vi "Size.vi"(8 "error in (no error)":errorcluster, 11 "Parameter to Hardware Map in":refnum<class "Parameter to Hardware Map.lvclass">) -> (0 "error out":errorcluster, 2 "Size":i32, 3 "Parameter to Hardware Map out":refnum<class "Parameter to Hardware Map.lvclass">)   [LabVIEW 2020, in "RxnRover.lvlib" / "Parameter to Hardware Map.lvclass"]
doc: "Return the size of the map."
uses:
  Parameter to Hardware Map.lvclass
  Parameter to Hardware Map.lvclass/Parameter to Hardware Map.ctl
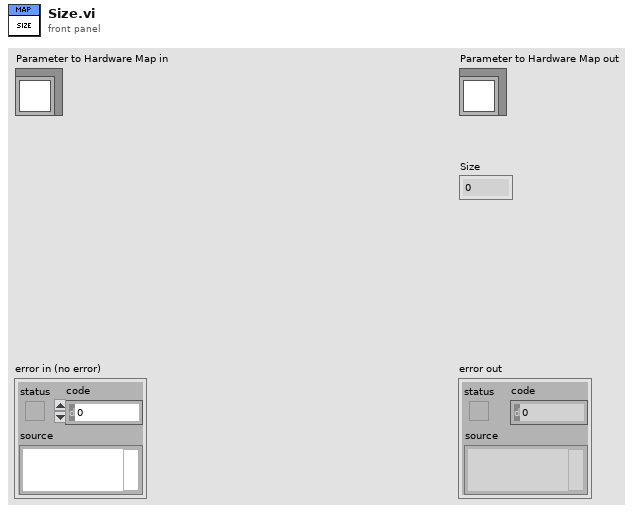
[diagram p1: front panel]
types:
  T1 = typedef "RxnRover.lvlib/Parameter to Hardware Map.lvclass/Pair.ctl" = cluster{"key":string, "values":refnum<class "Generic Plugin.lvclass">[]}
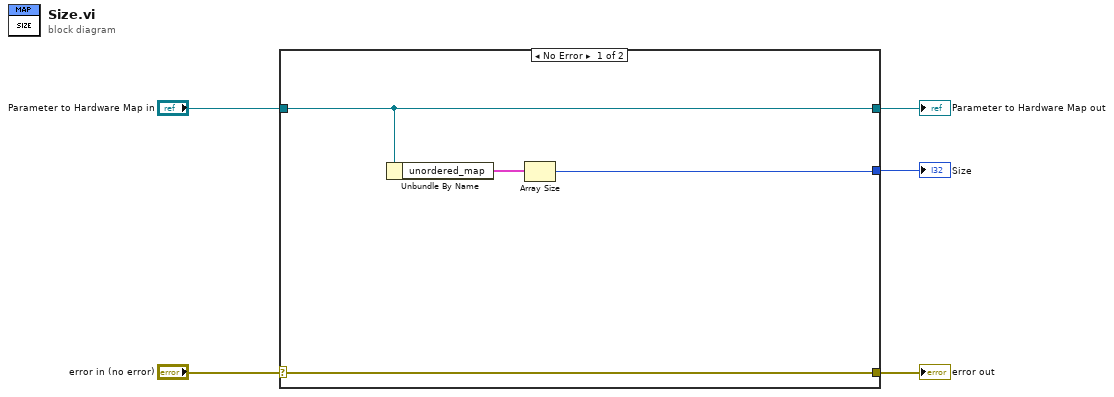
[diagram p0: block diagram]
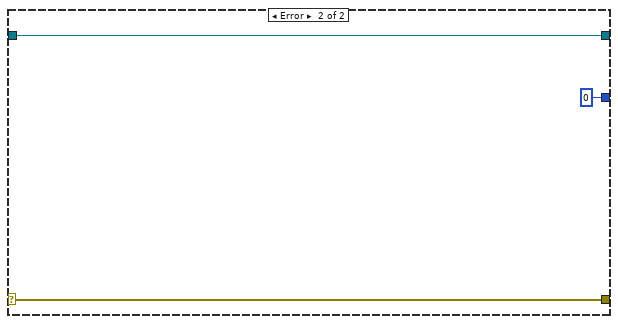
[diagram p2: hidden frame]
diagram:
  n1 = case shown="No Error" "error in (no error)" {
    selector: "error in (no error)" -> [w9 w12]
    tunnel: [w9 w12] -> w4
    tunnel: [w8 w11] -> w2
    tunnel: "Parameter to Hardware Map in" -> [w8 w11]
    tunnel: [w6 0] -> w1
    frame No Error {
      n2 = Unbundle By Name(w8) -> ("unordered_map"=w7:T1[])
      n3 = Array Size(array=w7) -> (size(s)=w6:i32)
    }
    frame Error {
    }
  }
  "error out" <- w4
  "Parameter to Hardware Map out" <- w2
  "Size" <- w1
